vi "GetStringBoundWithSpecifiedFont.vi"(8 "string":string, 9 "font":cluster{"name":string, "size":i16, "color":u32}, 10 "underline? (F)":bool) -> (11 "bounds":cluster{"width":u32, "height":u32})   [LabVIEW 2009, in "text.lvclass"]
uses:
  text.lvclass
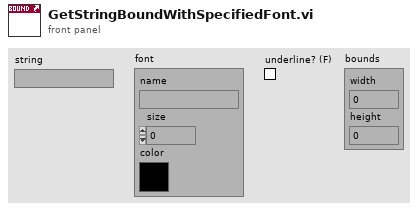
[diagram p1: front panel]
types:
  T1 = enum16{"User-specified Font", "Application Font", "System Font", "Dialog Font"}
  T2 = cluster{"Font Name:":string, "Size":i16, "Strikeout?":bool, "Italic?":bool, "Underline?":bool, "Outline?":bool, "Shadow?":bool, "Bold?":bool}
  T3 = cluster{"left":i16, "top":i16, "right":i16, "bottom":i16}
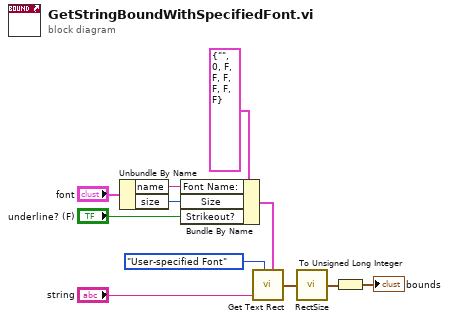
[diagram p0: block diagram]
diagram:
  n1 = Unbundle By Name("font") -> ("name"=w9:string, "size"=w8:i16)
  n2 = Bundle By Name(cluster=T2 {"Font Name:"="", "Size"=0, "Strikeout?"=FALSE, "Italic?"=FALSE, "Underline?"=FALSE, "Outline?"=FALSE, "Shadow?"=FALSE, "Bold?"=FALSE} ("[user-specified font]"), "Font Name:"=w9, "Size"=w8, "Strikeout?"="underline? (F)") -> (w5:T2)
  n3 = call <vilib>:"Get Text Rect.vi"("desired font(Application)"=T1."User-specified Font", "text"="string", "[user-specified font]"=w5) -> ("rect"=w6:T3)  [unwired: 6 in]
  n4 = call <vilib>:"RectSize.vi"("rect"=w6) -> ("point"=w2:cluster{"x":i16, "y":i16})
  n5 = To Unsigned Long Integer(number=w2) -> (unsigned 32bit integer=→"bounds":cluster{"x":u32, "y":u32})
